vi "0005_FireAtSpecificMinutesEveryWednesday.vi"(8 "error in (no error)":errorcluster) -> (0 "error out":errorcluster)   [LabVIEW 2013]
uses:
  <vilib>/addons/_JKI Toolkits/Caraya/classes/Assert/Assert True.vi
  <vilib>/addons/_JKI Toolkits/Caraya/classes/Test/Test.lvclass
  <vilib>/addons/_JKI Toolkits/Caraya/classes/Assert/Assert.lvclass
  source/openCron.lvlib
panel:
  out "after current month":timestamp
  out "Occurences":timestamp[](array[timestamp])
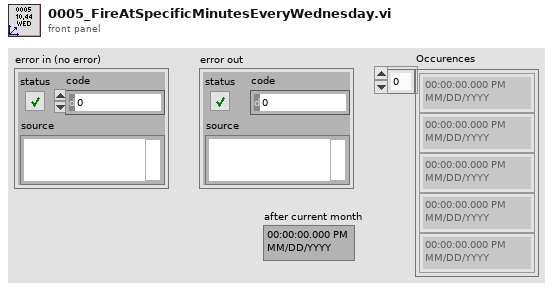
[diagram p1: front panel]
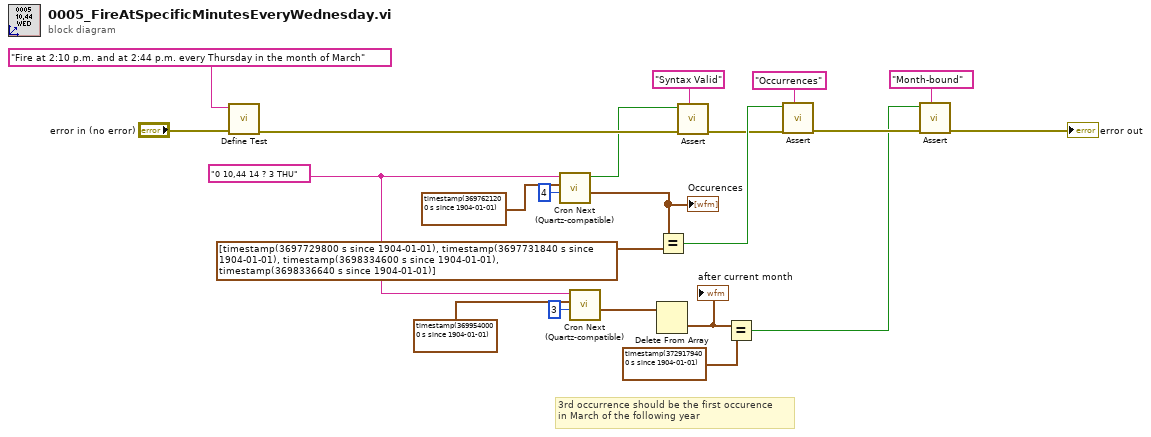
[diagram p0: block diagram]
diagram:
  w7 = "0 10,44 14 ? 3 THU" ("Expression")
  # "3rd occurrence should be the first occurence\nin March of the following year"
  n1 = call <vilib>:"Define Test.vi"("error in (no error)"="error in (no error)", "Label (VI Title)"="Fire at 2:10 p.m. and at 2:44 p.m. every Thursday in the month of March") -> ("error out"=w19:errorcluster)  [unwired: 9 in]
  n2 = call "Cron Next (Quartz-compatible).vi"("Nb Occurences (min: 1)"=u16 4, "Reference timestamp (Now)"=timestamp(3697621200 s since 1904-01-01) ("y"), "Cron Expression"=w7) -> ("Occurences"=w15:timestamp[], "syntax valid?"=w16:bool)  [unwired: 6 in, 1 out]
  "Occurences" <- w15
  n3 = call "Cron Next (Quartz-compatible).vi"("Nb Occurences (min: 1)"=u16 3, "Reference timestamp (Now)"=timestamp(3699540000 s since 1904-01-01) ("y"), "Cron Expression"=w7) -> ("Occurences"=w2:timestamp[])  [unwired: 6 in, 2 out]
  n4 = Delete From Array(array=w2) -> (deleted portion=w1:timestamp)  [unwired: 2 in, 1 out]
  "after current month" <- w1
  n5 = Equal?(x=w15, y=timestamp[] [timestamp(3697729800 s since 1904-01-01), timestamp(3697731840 s since 1904-01-01), timestamp(3698334600 s since 1904-01-01), timestamp(3698336640 s since 1904-01-01)]) -> (x = y?=w18:bool)
  n6 = call-poly <vilib>:"Assert.vi"("Label"="Syntax Valid" ("Label (VI Title)"), "error in (no error)"=w19, "True?"=w16) -> ("error out"=w17:errorcluster)  [unwired: 8 in]
  n7 = Equal?(x=w1, y=timestamp(3729179400 s since 1904-01-01)) -> (x = y?=w4:bool)
  n8 = call-poly <vilib>:"Assert.vi"("Label"="Occurrences" ("Label (VI Title)"), "error in (no error)"=w17, "True?"=w18) -> ("error out"=w9:errorcluster)  [unwired: 8 in]
  n9 = call-poly <vilib>:"Assert.vi"("Label"="Month-bound" ("Label (VI Title)"), "error in (no error)"=w9, "True?"=w4) -> ("error out"=→"error out":errorcluster)  [unwired: 8 in]
